vi "Magnetic_FIeld over Temp.vi"() -> ()   [LabVIEW 2020]
panel:
  out "Offset Check":bool
  out "Noise Check":bool
  out "Sensitivity Check":bool
  out "Z mean 0 offset":dbl[](array[numeric])
  out "Z std dev (noise)":dbl[](array[numeric])
  out "Z sensitivity LSB/mT":dbl[](array[numeric])
  in  "Choose Coil":string(combo)="Z"
  in  "Thermostream":refnum<visa-resource-name>="GPIB0::11::INSTR"
  out "error out":errorcluster
  in  "Multimetru":refnum<visa-resource-name>="GPIB0::24::INSTR"
  in  "SMU":refnum<visa-resource-name>="GPIB0::1::INSTR"
  in  "error in (no error)":errorcluster
  in  "Temperaturi":dbl[](array[numeric])=[-40.0, 25.0, 80.0, 125.0]
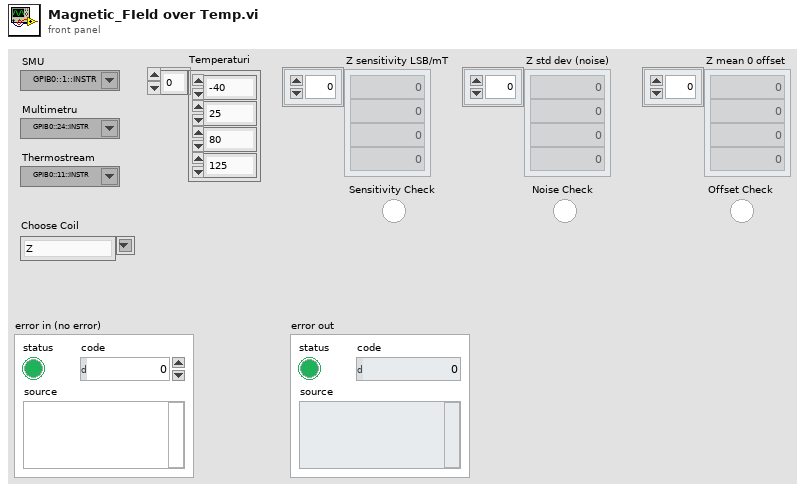
[diagram p1: front panel]
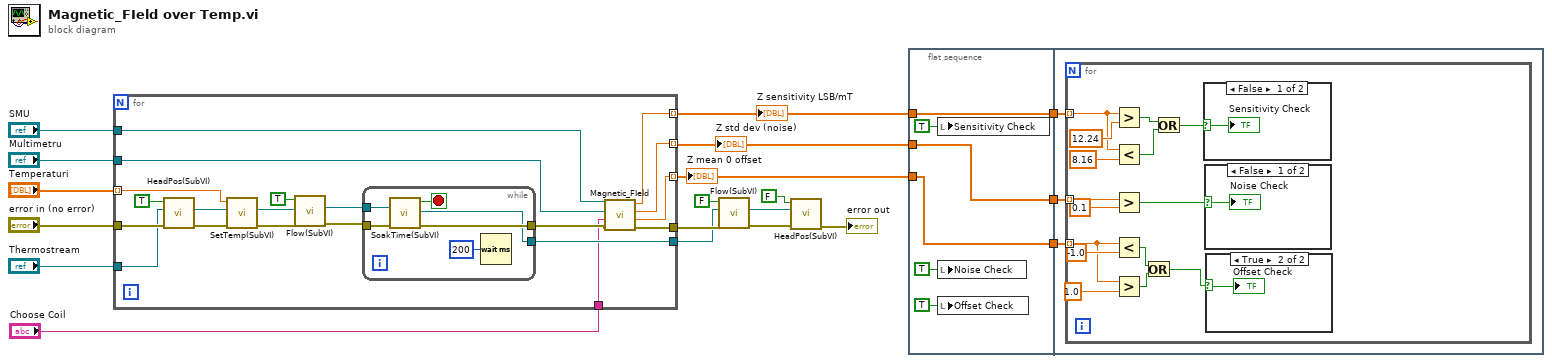
[diagram p0: block diagram]
diagram:
  n1 = for {
    tunnel: "Temperaturi" -> [w36] mode=indexing
    tunnel: "error in (no error)" -> [w39]
    tunnel: "SMU" -> [w27]
    tunnel: "Multimetru" -> [w26]
    tunnel: [w23] -> w14
    tunnel: "Thermostream" -> [w32]
    tunnel: [w28] -> w9
    tunnel: "Choose Coil" -> [w24]
    tunnel: [w22] -> w6 mode=indexing
    tunnel: [w21] -> w4 mode=indexing
    tunnel: [w20] -> w2 mode=indexing
    n2 = call "HeadPos(SubVI).vi"("error in (no error)"=w39, "VISA resource name"=w32, "Checkbox"=TRUE) -> ("error out"=w37:errorcluster, "VISA resource name 2"=w31:refnum<visa-resource-name>)  [unwired: 7 in]
    n3 = call "SetTemp(SubVI).vi"("error in (no error)"=w37, "VISA resource name"=w31, "Temp"=w36) -> ("error out"=w35:errorcluster, "VISA resource name out"=w30:refnum<visa-resource-name>)  [unwired: 7 in]
    n4 = call "Flow(SubVI).vi"("error in (no error)"=w35, "VISA resource name"=w30, "Flow state"=TRUE ("Checkbox")) -> ("error out"=w34:errorcluster, "VISA resource name 2"=w29:refnum<visa-resource-name>)  [unwired: 7 in]
    n5 = while {
      tunnel: [w43] -> w25
      tunnel: w34 -> [w44]
      tunnel: w29 -> [w41]
      tunnel: [w40] -> w28
      stop <- w42 stop-if-true
      n6 = call "SoakTime(SubVI).vi"("error in (no error)"=w44, "VISA resource name"=w41) -> ("error out"=w43:errorcluster, "VISA resource name out"=w40:refnum<visa-resource-name>, "soaked?"=w42:bool)  [unwired: 7 in]
      n7 = Wait (ms)(milliseconds to wait=u32 200) -> ()  [unwired: 1 out]
    }
    n8 = call "Magnetic_FIeld.vi"("error in (no error)"=w25, "Choose Coil"=w24, "SMU"=w26, "Power Supply"=w27) -> ("error out"=w23:errorcluster, "Z mean 0 (Offset)"=w20:dbl, "Z std dev"=w21:dbl, "Z Sensitivity LSB/mT"=w22:dbl)  [unwired: 4 in]
  }
  "Z sensitivity LSB/mT" <- w6
  "Z std dev (noise)" <- w4
  "Z mean 0 offset" <- w2
  n9 = call "Flow(SubVI).vi"("error in (no error)"=w14, "VISA resource name"=w9, "Flow state"=FALSE ("Checkbox")) -> ("error out"=w13:errorcluster, "VISA resource name 2"=w8:refnum<visa-resource-name>)  [unwired: 7 in]
  n10 = call "HeadPos(SubVI).vi"("error in (no error)"=w13, "VISA resource name"=w8, "Checkbox"=FALSE) -> ("error out"=→"error out":errorcluster)  [unwired: 7 in, 1 out]
  n11 = flat-sequence {
    tunnel: w6 -> [w51]
    tunnel: [w51] -> w5
    tunnel: w4 -> [w47]
    tunnel: [w47] -> w3
    tunnel: w2 -> [w46]
    tunnel: [w46] -> w1
    tunnel: w5 -> [w54]
    tunnel: w3 -> [w53]
    tunnel: w1 -> [w52]
    frame #0 {
      n12 = local write "Sensitivity Check"(TRUE ("Sensitivity Check")) -> ()
      n13 = local write "Noise Check"(TRUE ("Noise Check")) -> ()
      n14 = local write "Offset Check"(TRUE ("Offset Check")) -> ()
    }
    frame #1 {
      n15 = for {
        tunnel: w54 -> [w67] mode=indexing
        tunnel: w53 -> [w63] mode=indexing
        tunnel: w52 -> [w59] mode=indexing
        n16 = Greater?(x=w67, y=12.24) -> (0:w68:bool)
        n17 = Less?(x=w67, y=8.16) -> (x < y?=w65:bool)
        n18 = Greater?(x=w63, y=0.1) -> (0:w61:bool)
        n19 = Less?(x=w59, y=-1.0) -> (x < y?=w57:bool)
        n20 = Greater?(x=w59, y=1.0) -> (0:w56:bool)
        n21 = Or(x=w57, y=w56) -> (x .or. y?=w55:bool)
        n22 = Or(x=w68, y=w65) -> (x .or. y?=w64:bool)
        n23 = case shown="False" w64 {
          selector: w64 -> [w72 _]
          frame False {
            "Sensitivity Check" <- w72
          }
          frame True {
          }
        }
        n24 = case shown="False" w61 {
          selector: w61 -> [w71 _]
          frame False {
            "Noise Check" <- w71
          }
          frame True {
          }
        }
        n25 = case shown="True" w55 {
          selector: w55 -> [_ w70]
          frame False {
          }
          frame True {
            "Offset Check" <- w70
          }
        }
      }
    }
  }
